vi "json Clone - array path.vi"(8 "error in (no error)":errorcluster, 10 "path":string[](array[string]), 11 "JSON Document in":refnum<class "JSON Document.lvclass">) -> (0 "error out":errorcluster, 1 "JSON Document out":refnum<class "JSON Document.lvclass">, 3 "JSON Document out":refnum<class "JSON Document.lvclass">)   [LabVIEW 2015, in "JSON Document.lvclass"]
uses:
  JSON Document.lvclass
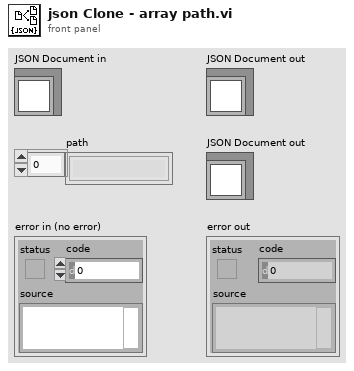
[diagram p1: front panel]
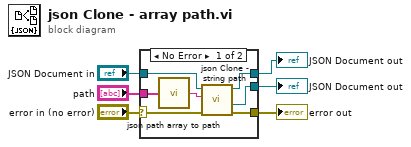
[diagram p0: block diagram]
diagram:
  n1 = case shown="No Error" "error in (no error)" {
    selector: "error in (no error)" -> [w11 w15]
    tunnel: [w10 w15] -> w5
    tunnel: [w12 w14] -> w3
    tunnel: "JSON Document in" -> [w13 w14]
    tunnel: "path" -> [w8 _]
    tunnel: [w9 _] -> w1
    frame No Error {
      n2 = call "json path array to path.vi"("path"=w8) -> ("String"=w7:string)
      n3 = call "json Clone - string path.vi"("error in (no error)"=w11, "path"=w7, "JSON Document in"=w13) -> ("error out"=w10:errorcluster, 1:"JSON Document out"=w9:refnum<class "JSON Document.lvclass">, 3:"JSON Document out"=w12:refnum<class "JSON Document.lvclass">)  [unwired: 6 in]
    }
    frame Error {
    }
  }
  "error out" <- w5
  "JSON Document out" <- w3
  "JSON Document out" <- w1
